vi "Read Array.vi"(8 "error in (no error)":errorcluster, 11 "JSON Array in":refnum<class "JSON Array.lvclass">) -> (0 "error out":errorcluster, 2 "Array":refnum<class "JSON Value.lvclass">[](array[class]), 3 "JSON Array out":refnum<class "JSON Array.lvclass">)   [LabVIEW 2020, in "Library Commun.lvlib" / "JSON Array.lvclass"]
uses:
  JSON Array.lvclass
  JSON Value/JSON Value.lvclass
  JSON Array.lvclass/JSON Array.ctl
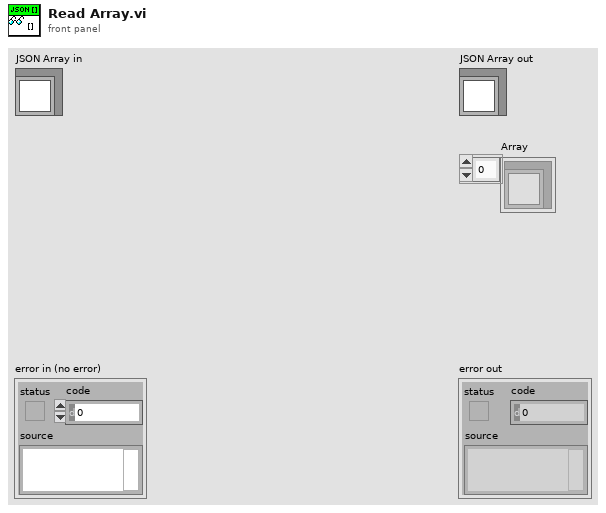
[diagram p1: front panel]
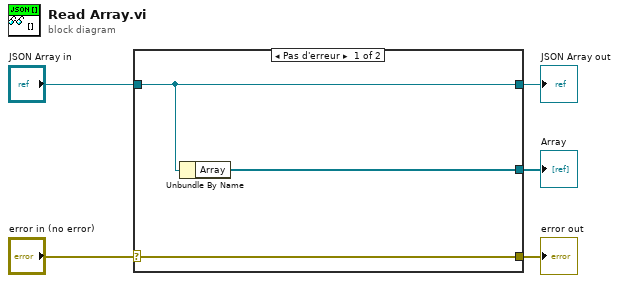
[diagram p0: block diagram]
diagram:
  n1 = case shown="Pas d'erreur" "error in (no error)" {
    selector: "error in (no error)" -> [w8 w9]
    tunnel: [w8 w9] -> w4
    tunnel: [w7 w10] -> w2
    tunnel: "JSON Array in" -> [w7 w10]
    tunnel: [w6 _] -> w1
    frame No Error {
      n2 = Unbundle By Name(w7) -> ("Array"=w6:refnum<class "JSON Value.lvclass">[])
    }
    frame Error {
    }
  }
  "error out" <- w4
  "JSON Array out" <- w2
  "Array" <- w1
